vi "Shooter_axl.vi"() -> (1 "Filtered z":dbl format="%0.2f", 2 "Filtered y":dbl format="%0.2f", 3 "Filtered x":dbl format="%0.2f")   [LabVIEW 2012]
uses:
  Program Files (x86)/National Instruments/LabVIEW 2012/examples/FRC/I2C/ADXL345 I2C/Driver/ADXL345 I2C Axis.ctl
  <vilib>/ptbypt/NI_PtbyPt.lvlib
panel:
  out "mean z":dbl format="%0.2f"
  out "mean y":dbl format="%0.2f"
  out "mean x":dbl format="%0.2f"
  out "z":dbl
  out "y":dbl
  out "x":dbl
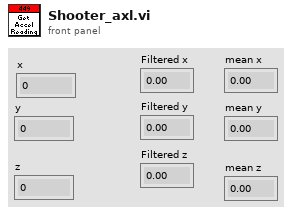
[diagram p1: front panel]
types:
  T1 = typedef "ADXL345 I2C Axis.ctl" = u8
  T2 = typedef "WPI_I2CDevRef.ctl" = cluster{"DevStatus":errorcluster, "Digital Module":T3, "Device Address":u8}
  T3 = typedef "FPGA_TypedefDigitalModule.ctl" = enum16{"Digital Module 1", "Digital Module 2"}
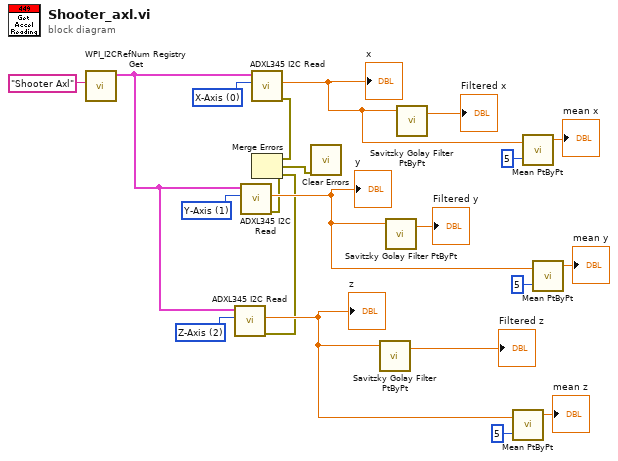
[diagram p0: block diagram]
diagram:
  w19 = T1 2 items=["X-Axis", "Y-Axis", "Z-Axis"] ("Axis")
  w20 = T1 1 items=["X-Axis", "Y-Axis", "Z-Axis"] ("Axis")
  w21 = T1 0 items=["X-Axis", "Y-Axis", "Z-Axis"] ("Axis")
  n1 = call <vilib>:"WPI_I2CRefNum Registry Get.vi"("refnum name"="Shooter Axl") -> ("I2CDevRef"=w18:T2)  [unwired: 9 in, 1 out]
  n2 = call "ADXL345 I2C Read.vi"("Axis"=w19, "I2CDevRef"=w18) -> ("error out"=w2:errorcluster, "Acceleration"=w6:dbl)  [unwired: 7 in, 1 out]
  "z" <- w6
  n3 = call "ADXL345 I2C Read.vi"("Axis"=w20, "I2CDevRef"=w18) -> ("error out"=w3:errorcluster, "Acceleration"=w5:dbl)  [unwired: 7 in, 1 out]
  "y" <- w5
  n4 = call "ADXL345 I2C Read.vi"("Axis"=w21, "I2CDevRef"=w18) -> ("error out"=w4:errorcluster, "Acceleration"=w11:dbl)  [unwired: 7 in, 1 out]
  "x" <- w11
  n5 = Merge Errors(w4, w3, w2) -> (w1:errorcluster)
  n6 = call <vilib>:"Clear Errors.vi"("error in (no error)"=w1) -> ()  [unwired: 6 in, 1 out]
  n7 = call <vilib>:"Savitzky Golay Filter PtByPt.vi"("x"=w6) -> ("Filtered x"=→"Filtered z":dbl)  [unwired: 3 in, 1 out]
  n8 = call <vilib>:"Savitzky Golay Filter PtByPt.vi"("x"=w5) -> ("Filtered x"=→"Filtered y":dbl)  [unwired: 3 in, 1 out]
  n9 = call <vilib>:"Savitzky Golay Filter PtByPt.vi"("x"=w11) -> ("Filtered x"=→"Filtered x":dbl)  [unwired: 3 in, 1 out]
  n10 = call <vilib>:"Mean PtByPt.vi"("x"=w6, "sample length"=5) -> ("mean"=→"mean z":dbl)  [unwired: 2 in, 1 out]
  n11 = call <vilib>:"Mean PtByPt.vi"("x"=w11, "sample length"=5) -> ("mean"=→"mean x":dbl)  [unwired: 2 in, 1 out]
  n12 = call <vilib>:"Mean PtByPt.vi"("x"=w5, "sample length"=5) -> ("mean"=→"mean y":dbl)  [unwired: 2 in, 1 out]
